vi "Index Point Calibration.vi"(8 "error in (no error)":errorcluster caption="错误输入（无错误）", 10 "kOffsInitRef":i32, 11 "asicHandle":i32) -> (0 "error out":errorcluster caption="错误输出", 2 "kOffsInitRef out":i32, 3 "function return":i32)   [LabVIEW 2018]
doc: "extern int __stdcall APSxIndexPointCalibration (int asicHandle, OUT int * kOffsInitRef);"
uses:
  APSx.dll/APSx.dll
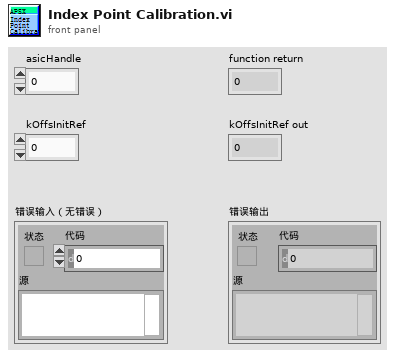
[diagram p1: front panel]
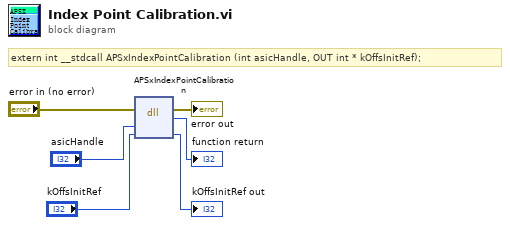
[diagram p0: block diagram]
diagram:
  # "extern int __stdcall APSxIndexPointCalibration (int asicHandle, OUT int * kOffsInitRef);"
  n1 = dll-call lib="PTH2[abs D项目Feng恒隆项目Labview传感器对中台SourcesAPSx.dllAPSx.*" fn="APSxIndexPointCalibration"(error in="error in (no error)", "asicHandle"="asicHandle", "kOffsInitRef"="kOffsInitRef") -> (error out=→"error out":errorcluster, →"function return":i32, "kOffsInitRef"=→"kOffsInitRef out":i32)  [unwired: 3 in, 1 out]
